vi "G4BaseTemplate_Simple_5x6x5_SetProperty.vi"(0 "reference in":refnum<class "G4BaseTemplate_Simple_5x6x5.lvclass">, 7 "Property":dbl, 11 "Error In":errorcluster) -> (4 "reference out":refnum<class "G4BaseTemplate_Simple_5x6x5.lvclass">, 15 "Error Out":errorcluster)   [LabVIEW 2020]
uses:
  <resource>/Framework/Providers/Open_GDS/ClassProviders/Provider_EndevoGOOP400/Templates/G4BaseTemplate_Simple_5x6x5/G4BaseTemplate_Simple_5x6x5.lvclass
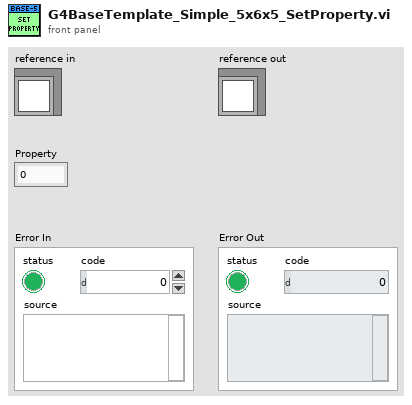
[diagram p1: front panel]
types:
  T1 = typedef "G4BaseTemplate_Simple_5x6x5.lvclass/ObjectAttributes.ctl" = cluster{"Attribute1":dbl}
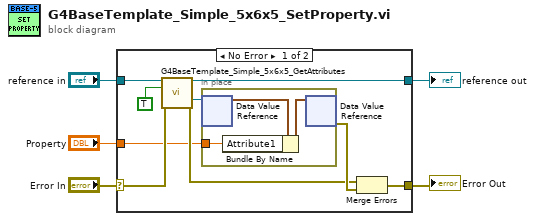
[diagram p0: block diagram]
diagram:
  n1 = case shown="No Error" "Error In" {
    selector: "Error In" -> [w12 w19]
    tunnel: [w7 w19] -> w4
    tunnel: [w13 w18] -> w2
    tunnel: "reference in" -> [w14 w18]
    tunnel: "Property" -> [w6 _]
    frame No Error {
      n2 = call <resource>:"G4BaseTemplate_Simple_5x6x5_GetAttributes.vi"("reference in"=w14, "OnlyGetDvrReference(False)"=TRUE, "error in (no error)"=w12) -> ("reference out"=w13:refnum<class "G4BaseTemplate_Simple_5x6x5.lvclass">, "DataRef"=w9:refnum<data-value>, "error out"=w8:errorcluster)  [unwired: 9 in, 1 out]
      n3 = in-place {
        in-place-border: w6 -> [w17]
        n4 = in-place-dvr #1(w9) -> (w16:T1)  [unwired: 1 out]
        n5 = Bundle By Name(cluster=w16, "Attribute1"=w17) -> (w15:T1)
        n6 = in-place-dvr #1(w15) -> (w10:errorcluster)  [unwired: 1 out]
      }
      n7 = Merge Errors(w8, w10) -> (w7:errorcluster)
    }
    frame Error {
    }
  }
  "Error Out" <- w4
  "reference out" <- w2
